vi "XLP80_FGlob_ResetAlarm.vi"(8 "err in":errorcluster caption="error") -> (0 "err out":errorcluster caption="error")   [LabVIEW 2021]
uses:
  1886_FGlob_TDefs_Enum_FGlobItems.ctl
  XLP80_General_Libs/Kirschenhofer_Libs/KH Turck EthernetIP 17.12/KH TURCK TypeDefs FGlob.ctl
  XLP80_Globals/XLP80_Globals_Status.vi
  XLP80_Globals/Globals_Settings_XLP80.vi
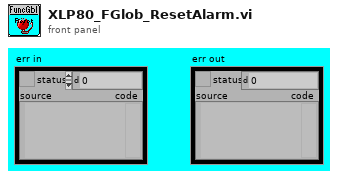
[diagram p1: front panel]
types:
  T1 = typedef "KH TURCK TypeDefs FGlob.ctl" = enum16{"Put one", "Put all", "Recall one", "Recall all"}
  T2 = typedef "1886_FGlob_TDefs_Enum_FGlobItems.ctl" = enum16{"Put one", "Put all", "Recall one", "Recall all"}
  T3 = typedef "XLP80_Action_TDefEnumControl.ctl" = enum16{"Testmode_A", "Testmode_B"}
  T4 = typedef "KH_DAQ_TypeDefs_Cluster AO.ctl" = cluster{"Signal Name":string[], "Description":string[], "Phys Unit":string[], "Messbereich":T5[], "Chan":u16[], "Phys Min":sgl[], "Phys Max":sgl[], "Offset":sgl[], "Nr":u16[], "SensorType 2":T6[], "Bereich":T7[], "Default":sgl[]}
  T5 = typedef "KH_DAQ_TypeDefs_Messbereich.ctl" = enum16{"-10V ... +10V", "0V ... +10V", "+2V ... +10V", "0V ... +5V", "+1V ... +5V", "-1V ... +1V", "-500mV ... +500mV", "-100mV ... +100mV", "-50mV ... +50mV", "0mA ... +20mA", "+4mA ... +20mA", "-20mA ... +20mA", "0 Ohm ... 100 Ohm", "0 Ohm ... 400 Ohm", "0 Ohm ... 2000 Ohm", "0 Ohm ... 4000 Ohm", "-200°C ... 150°C PT100", "-200°C ... 150°C PT200", "-200°C ... 150°C PT500", "-200°C ... 150°C PT1000", "-60°C ... 150°C Ni100", "-60°C ... 150°C Ni1000", "-200°C ... 850°C PT100", "-200°C ... 850°C PT200", "-200°C ... 850°C PT500", "-200°C ... 850°C PT1000", "-50°C ... 250°C Ni100", "-50°C ... 250° Ni 1000"}
  T6 = typedef "KH EthernetIPConfig TypeDefs ModuleTyp.ctl" = enum16{"TBEN-S2-4AI", "TBEN-S1-8DXP", "TBEN-S2-2RFID-4DXP", "TBEN-S2-4AO", "TBEN-S2-4IOL"}
  T7 = typedef "KH_DAQ_TypeDefs_Bereich.ctl" = enum16{"Standard", "extended Range", "NE43", ""}
  T8 = cluster{"Signal Name":string[], "Description":string[], "Unit":string[], "Default":dbl[], "Min":dbl[], "Max":dbl[], "Preconditions":bool[], "HV & Software":bool[], "Basis Funktion":bool[], "Power Management":bool[], "OperationMode":bool[], "Shutdown":bool[], "Alarm":bool[], "LogEnable":bool[]}
  T9 = cluster{"Signal Name":string[], "Description":string[], "Unit":string[], "Default":dbl[], "Min":dbl[], "Max":dbl[], "TestmodeA":bool[], "LogEnable":bool[]}
  T10 = typedef "KH_DAQ_TURCK_TypeDefs_Cluster DO.ctl" = cluster{"Def":bool[], "Signal Name":string[], "Description":string[], "Chan":u16[], "Inv":bool[], "Nr":u16[], "SensorType":T6[]}
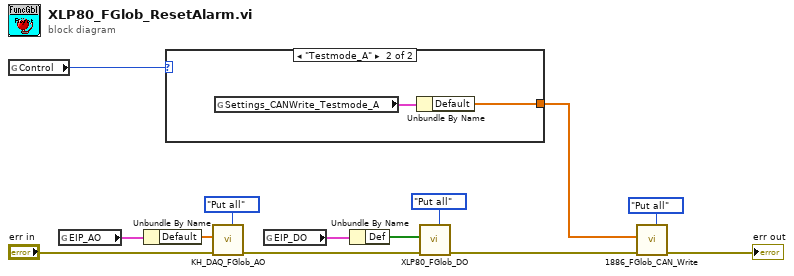
[diagram p0: block diagram]
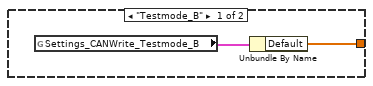
[diagram p2: hidden frame]
diagram:
  n1 = global read "XLP80_Globals_Status.vi" "Control"() -> (w12:T3)
  n2 = global read "Globals_Settings_XLP80.vi" "EIP_AO"() -> (w5:T4)
  n3 = Unbundle By Name(w5) -> ("Default"=w4:sgl[])
  n4 = case shown="\"Testmode_A\"" w12 {
    tunnel: [w14 w16] -> w11
    frame "Testmode_B" {
      n5 = global read "Globals_Settings_XLP80.vi" "Settings_CANWrite_Testmode_B"() -> (w15:T8)
      n6 = Unbundle By Name(w15) -> ("Default"=w14:dbl[])
    }
    frame "Testmode_A" {
      n7 = global read "Globals_Settings_XLP80.vi" "Settings_CANWrite_Testmode_A"() -> (w17:T9)
      n8 = Unbundle By Name(w17) -> ("Default"=w16:dbl[])
    }
  }
  n9 = call "KH_DAQ_FGlob_AO.vi"("Function (Recall One)"=KH_TURCK_TypeDefs_FGlob."Put all", "err in"="err in", "AO Values IN"=w4) -> ("err out"=w3:errorcluster)  [unwired: 6 in, 2 out]
  n10 = global read "Globals_Settings_XLP80.vi" "EIP_DO"() -> (w8:T10)
  n11 = Unbundle By Name(w8) -> ("Def"=w7:bool[])
  n12 = call "XLP80_FGlob_DO.vi"("Function (Set)"=1886_FGlob_TDefs_Enum_FGlobItems."Put all", "err in"=w3, "DXP Values IN"=w7) -> ("err out"=w6:errorcluster)  [unwired: 6 in, 2 out]
  n13 = call "1886_FGlob_CAN_Write.vi"("Function (Recall One)"=1886_FGlob_TDefs_Enum_FGlobItems."Put all", "err in"=w6, "AO Values IN"=w11) -> ("err out"=→"err out":errorcluster)  [unwired: 6 in, 2 out]
